vi "CRYStart Front Panel.vi"(11 "Vi Ref":refnum<vi>) -> ()   [LabVIEW 2013]
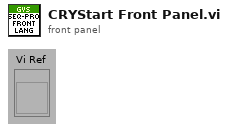
[diagram p1: front panel]
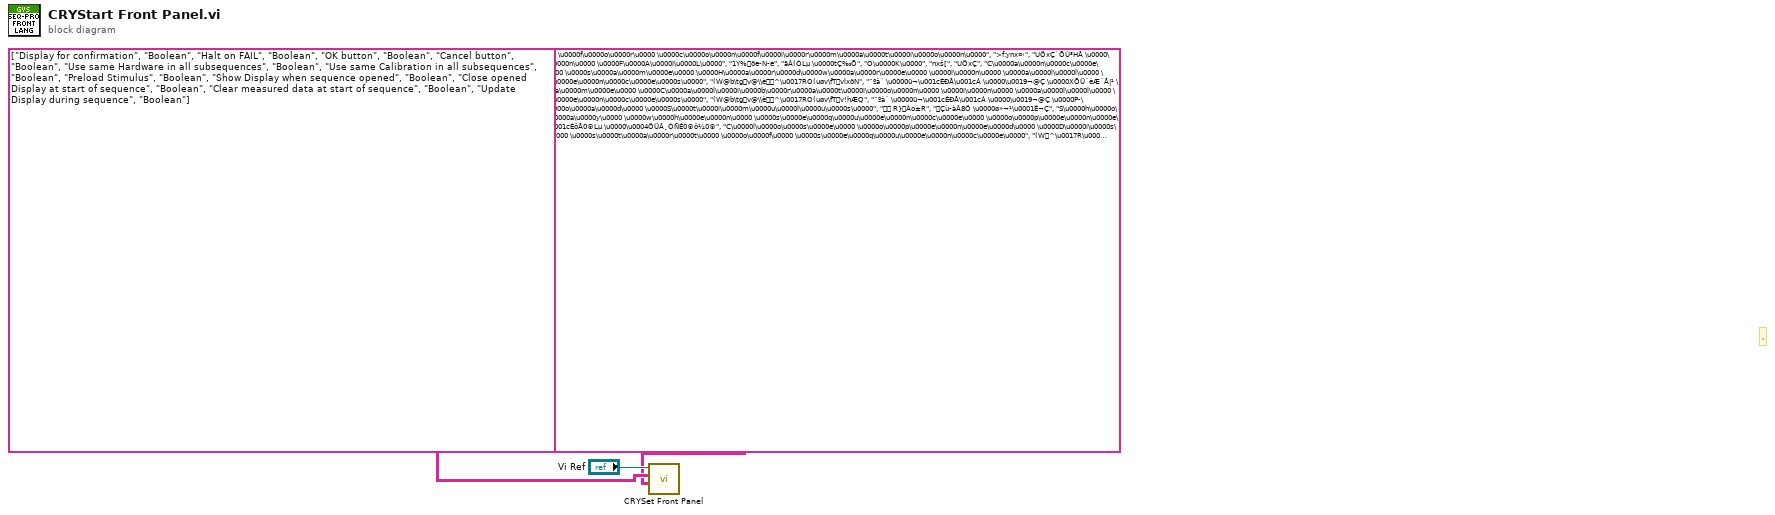
[diagram p0: block diagram]
diagram:
  # ","
  # "Caption, Tab Page, Multilist Header, Button 4"
  # "Control Type"
  # "Control Name and Tab"
  n1 = call "CRYSet Front Panel.vi"("Caption(Boolean Text)"=string[][] [["D\u0000i\u0000s\u0000p\u0000l\u0000a\u0000y\u0000 \u0000f\u0000o\u0000r\u0000 \u0000c\u0000o\u0000n\u0000f\u0000i\u0000r\u0000m\u0000a\u0000t\u0000i\u0000o\u0000n\u0000", ">f:ynx¤‹", "UÖxÇ`ÕÙ³HÅ \u0000\u0004ÖÜÂ"], ["H\u0000a\u0000l\u0000t\u0000 \u0000o\u0000n\u0000 \u0000F\u0000A\u0000I\u0000L\u0000", "1Y%öe-N­e", "äÂ(ÓLµ \u0000tÇ‰Õ"], ["O\u0000K\u0000", "nxš[", "UÖxÇ"], ["C\u0000a\u0000n\u0000c\u0000e\u0000l\u0000", "ÖSˆm", "èÍŒÁ"], ["U\u0000s\u0000e\u0000 \u0000s\u0000a\u0000m\u0000e\u0000 \u0000H\u0000a\u0000r\u0000d\u0000w\u0000a\u0000r\u0000e\u0000 \u0000i\u0000n\u0000 \u0000a\u0000l\u0000l\u0000 \u0000s\u0000u\u0000b\u0000s\u0000e\u0000q\u0000u\u0000e\u0000n\u0000c\u0000e\u0000s\u0000", "(W@b\tgv@\\è^\u0017RO(uøv\fTvlxöN", "¨ºà´ \u0000ü¬\u001cÈÐÅ\u001cÁ \u0000\u0019¬@Ç \u0000XÕÜ´èÆ´Å|¹ \u0000¬À©Æ"], ["U\u0000s\u0000e\u0000 \u0000s\u0000a\u0000m\u0000e\u0000 \u0000C\u0000a\u0000l\u0000i\u0000b\u0000r\u0000a\u0000t\u0000i\u0000o\u0000n\u0000 \u0000i\u0000n\u0000 \u0000a\u0000l\u0000l\u0000 \u0000s\u0000u\u0000b\u0000s\u0000e\u0000q\u0000u\u0000e\u0000n\u0000c\u0000e\u0000s\u0000", "(W@b\tgv@\\è^\u0017RO(uøv\fTv!hÆQ", "¨ºà´ \u0000ü¬\u001cÈÐÅ\u001cÁ \u0000\u0019¬@Ç \u0000P­\u0000ÉDÇ \u0000¬À©Æ"], ["P\u0000r\u0000e\u0000l\u0000o\u0000a\u0000d\u0000 \u0000S\u0000t\u0000i\u0000m\u0000u\u0000l\u0000u\u0000s\u0000", " R}Ào±R", "Çù­àÂ8Ö \u0000ø»¬¹\u0001È¬Ç"], ["S\u0000h\u0000o\u0000w\u0000 \u0000D\u0000i\u0000s\u0000p\u0000l\u0000a\u0000y\u0000 \u0000w\u0000h\u0000e\u0000n\u0000 \u0000s\u0000e\u0000q\u0000u\u0000e\u0000n\u0000c\u0000e\u0000 \u0000o\u0000p\u0000e\u0000n\u0000e\u0000d\u0000", "S_^\u0017RSb\u0000_öe>f:y", "ü¬\u001cÈôÅ0®Lµ \u0000\u0004ÖÜÂ¸ÓÑÉ0®ô¼0®"], ["C\u0000l\u0000o\u0000s\u0000e\u0000 \u0000o\u0000p\u0000e\u0000n\u0000e\u0000d\u0000 \u0000D\u0000i\u0000s\u0000p\u0000l\u0000a\u0000y\u0000 \u0000a\u0000t\u0000 \u0000s\u0000t\u0000a\u0000r\u0000t\u0000 \u0000o\u0000f\u0000 \u0000s\u0000e\u0000q\u0000u\u0000e\u0000n\u0000c\u0000e\u0000", "(W^\u0017R\u0000_ËYöesQíSb\u0000_>f:yek¤", "ü¬\u001cÈäÂ‰ÕÜÂ‘ÇLµ \u0000ôÅ$¸ÄÉ \u0000\u0004ÖÜÂ¸ÓÑÉ0® \u0000ë²0®"], ["C\u0000l\u0000e\u0000a\u0000r\u0000 \u0000m\u0000e\u0000a\u0000s\u0000u\u0000r\u0000e\u0000d\u0000 \u0000d\u0000a\u0000t\u0000a\u0000 \u0000a\u0000t\u0000 \u0000s\u0000t\u0000a\u0000r\u0000t\u0000 \u0000o\u0000f\u0000 \u0000s\u0000e\u0000q\u0000u\u0000e\u0000n\u0000c\u0000e\u0000", "(W^\u0017R\u0000_ËYöe\u0005ndKmÕpenc", "ü¬\u001cÈäÂÕÜÂÇLµ \u0000!Î\u0015È\u001c´ \u0000ÇÌ¸ \u0000ÀÉ°Æ0®"], ["U\u0000p\u0000d\u0000a\u0000t\u0000e\u0000 \u0000D\u0000i\u0000s\u0000p\u0000l\u0000a\u0000y\u0000 \u0000d\u0000u\u0000r\u0000i\u0000n\u0000g\u0000 \u0000s\u0000e\u0000q\u0000u\u0000e\u0000n\u0000c\u0000e\u0000", "(WÐL^\u0017R-Nôf°e>f:yek¤", "ü¬\u001cÈäÂ‰Õü¬\u0015ÈÐÅ \u0000\u0004ÖÜÂ¸ÓÑÉ0® \u00001¬àÂ"]], "Control ID and Type(Label Name, Type)"=string[][] [["Display for confirmation", "Boolean"], ["Halt on FAIL", "Boolean"], ["OK button", "Boolean"], ["Cancel button", "Boolean"], ["Use same Hardware in all subsequences", "Boolean"], ["Use same Calibration in all subsequences", "Boolean"], ["Preload Stimulus", "Boolean"], ["Show Display when sequence opened", "Boolean"], ["Close opened Display at start of sequence", "Boolean"], ["Clear measured data at start of sequence", "Boolean"], ["Update Display during sequence", "Boolean"]], "Vi Ref"="Vi Ref") -> ()  [unwired: 9 in]
